vi "Post.vi"(0 "InfluxDB Client in":refnum<class "Client.lvclass">, 5 "Query":T1, 9 "buffer":string, 11 "error in (no error)":errorcluster) -> (4 "InfluxDB Client out":refnum<class "Client.lvclass">, 6 "body":string, 8 "Status code":string, 10 "Headers":T1, 15 "error out":errorcluster)   [LabVIEW 2018, in "InfluxDB Client.lvlib" / "Client.lvclass"]
uses:
  Client.lvclass
  <userlib>/_OpenG.lib/dictionary/dictionary.llb/Dictionary Object RefNum__ogtk.ctl
  <userlib>/_OpenG.lib/dictionary/dictionary.llb/Dictionary Object RefNum - Enum__ogtk.ctl
  Client.lvclass/Client.ctl
  <vilib>/httpClient/POSTBuffer.vi
  <vilib>/httpClient/LabVIEWHTTPClient.lvlib
panel:
  out "query":string
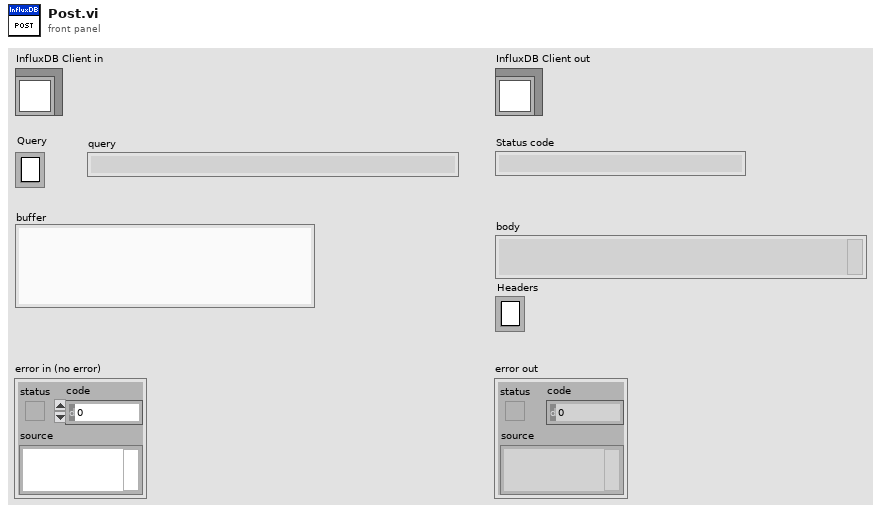
[diagram p1: front panel]
types:
  T1 = typedef "Dictionary Object RefNum__ogtk.ctl" = refnum<k1>
  T2 = typedef "LabVIEWHTTPClient.lvlib/ClientHandle.ctl" = refnum<k1>
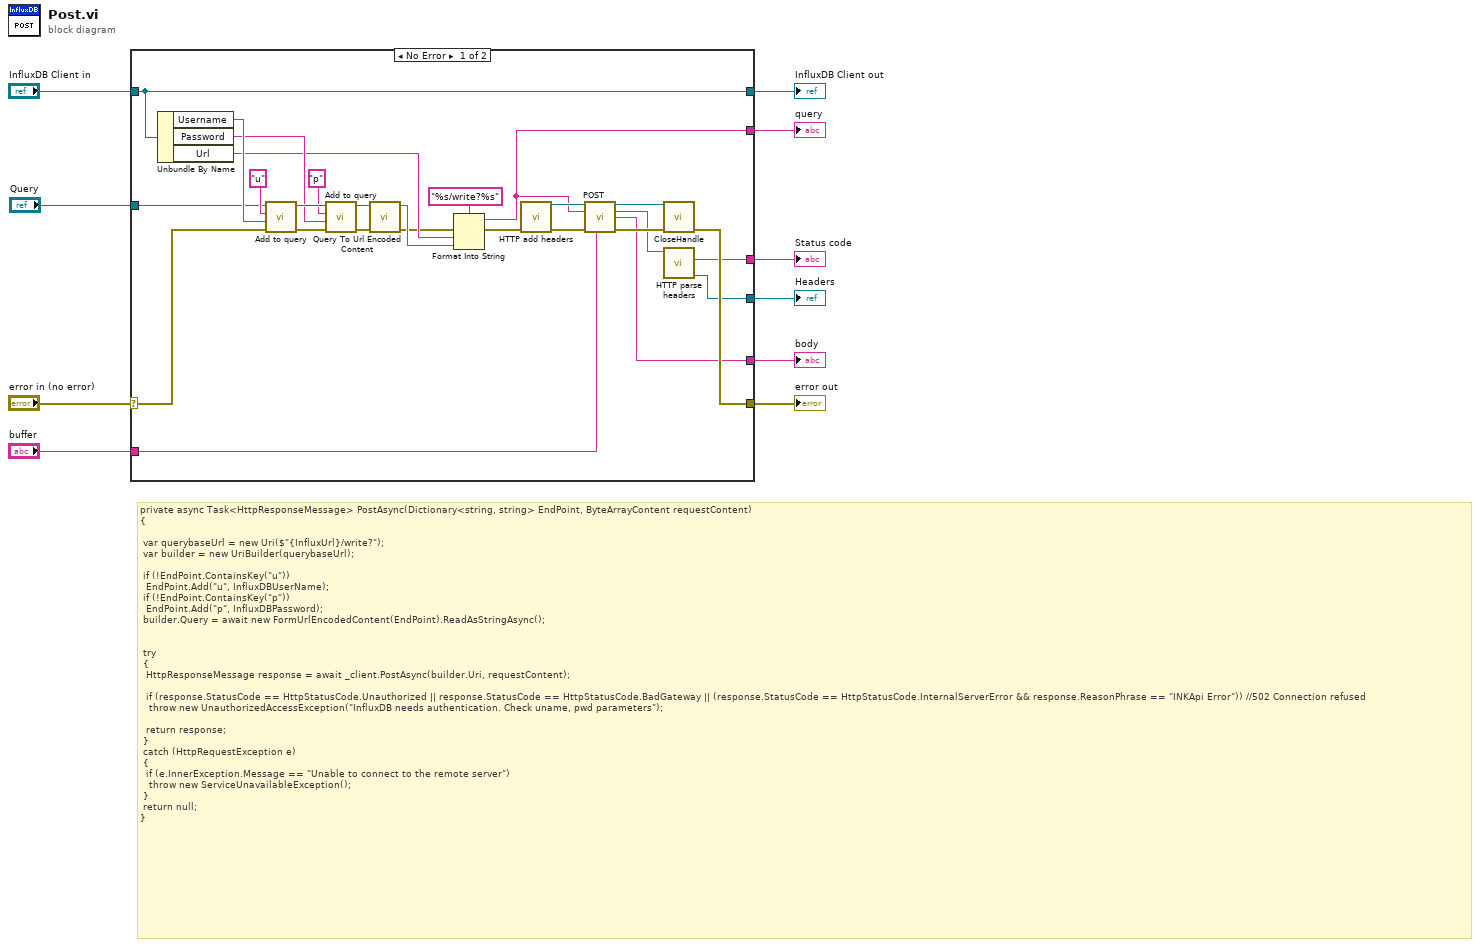
[diagram p0: block diagram]
diagram:
  # "private async Task<HttpResponseMessage> PostAsync(Dictionary<string, string> EndPoint, ByteArrayContent requestContent)\n{\n\n\tvar querybaseUrl = new Uri($\"{InfluxUrl}/write?\");\n\tvar builder = new UriBuilder(querybaseUrl);\n\n\tif (!EndPoint.ContainsKey(\"u\"))\n\t\tEndPoint.Add(\"u\", InfluxDBUserName);\n\tif (!EndPoint.ContainsKey(\"p\"))\n\t\tEndPoint.Add(\"p\", InfluxDBPassword);\n\tbuilder.Query = await new FormUrlEncodedContent(EndPoint).ReadAsStringAsync();\n\n\n\ttry\n\t{\n\t\tHttpResponseMessage response = await _client.PostAsync(builder.Uri, requestContent);\n\n\t\tif (response.StatusCode == HttpStatusCode.Unauthorized || response.StatusCode == HttpStatusCode.BadGateway || (response.StatusCode == HttpStatusCode.InternalServerError && response.ReasonPhrase == \"INKApi Error\")) //502 Connection refused\n\t\t\tthrow new UnauthorizedAccessException(\"InfluxDB needs authentication. Check uname, pwd parameters\");\n\n\t\treturn response;\n\t}\n\tcatch (HttpRequestException e)\n\t{\n\t\tif (e.InnerException.Message == \"Unable to connect to the remote server\")\n\t\t\tthrow new ServiceUnavailableException();\n\t}\n\treturn null;\n}"
  n1 = case shown="No Error" "error in (no error)" {
    selector: "error in (no error)" -> [w16 w39]
    tunnel: [w22 w39] -> w9
    tunnel: [w37 w38] -> w7
    tunnel: "InfluxDB Client in" -> [w37 w38]
    tunnel: "Query" -> [w20 _]
    tunnel: "buffer" -> [w15 _]
    tunnel: [w14 _] -> w4
    tunnel: [w13 _] -> w3
    tunnel: [w12 _] -> w2
    tunnel: [w11 _] -> w1
    frame No Error {
      n2 = Unbundle By Name(w37) -> ("Username"=w35:string, "Password"=w32:string, "Url"=w24:string)
      n3 = call "Add to query.vi"("error in (no error)"=w16, "Value"=w35, "Parameter"="u", "Query in"=w20) -> ("error out"=w19:errorcluster, "Query out"=w34:T1)  [unwired: 6 in]
      n4 = call "Add to query.vi"("error in (no error)"=w19, "Value"=w32, "Parameter"="p", "Query in"=w34) -> ("error out"=w18:errorcluster, "Query out"=w21:T1)  [unwired: 6 in]
      n5 = call "Query To Url Encoded Content.vi"("error in (no error)"=w18, "Query"=w21) -> ("error out"=w17:errorcluster, "Url Encoded Content"=w23:string)  [unwired: 8 in]
      n6 = Format Into String(format string="%s/write?%s", error in=w17, w24, w23) -> (resulting string=w14:string, error out=w25:errorcluster)  [unwired: 1 in]
      n7 = call "HTTP add headers.vi"("error in (no error)"=w25) -> ("client handle out"=w27:T2, "error out"=w26:errorcluster)  [unwired: 13 in]
      n8 = call-poly <vilib>:"POST.vi"("client handle"=w27, "url"=w14, "buffer"=w15, "error in (no error)"=w26) -> ("client handle out"=w30:T2, "headers"=w28:string, "body"=w13:string, "error out"=w29:errorcluster)  [unwired: 8 in]
      n9 = call <vilib>:"CloseHandle.vi"("client handle"=w30, "error in (no error)"=w29) -> ("error out"=w22:errorcluster)  [unwired: 13 in]
      n10 = call "HTTP parse headers.vi"("HTTP headers"=w28) -> ("Headers out"=w12:T1, "Status code"=w11:string)  [unwired: 7 in, 2 out]
    }
    frame Error {
    }
  }
  "error out" <- w9
  "InfluxDB Client out" <- w7
  "query" <- w4
  "body" <- w3
  "Headers" <- w2
  "Status code" <- w1
